vi "BUFMGR_get_maxmem.vi"(11 "error in (no error)":errorcluster) -> (4 "return":u64 format="%.0x", 15 "error out":errorcluster)   [LabVIEW 2016]
uses:
  c/lib/libbuf.so
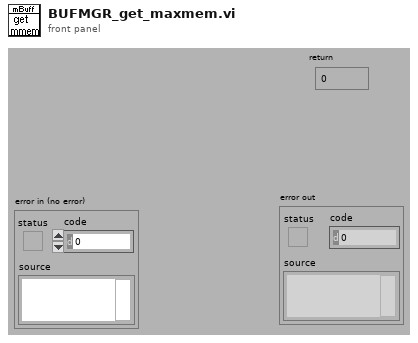
[diagram p1: front panel]
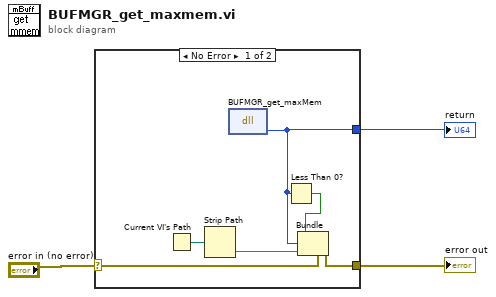
[diagram p0: block diagram]
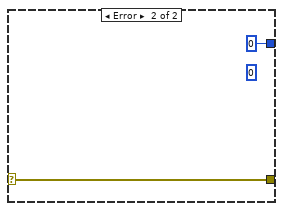
[diagram p2: hidden frame]
diagram:
  n1 = case shown="No Error" "error in (no error)" {
    selector: "error in (no error)" -> [w4 w10]
    tunnel: [w7 u32 0] -> w3
    tunnel: [w9 w10] -> w2
    frame No Error {
      n2 = Current VI's Path() -> (path=w6:path)
      n3 = Strip Path(path=w6) -> (name=w5:string)  [unwired: 1 out]
      n4 = dll-call lib="home/simager/panview/PAN/Modules/buffermgr/private/c/lib/libbuf.so" fn="BUFMGR_get_maxMem"() -> ("return type"=w7:u64)  [unwired: 3 in, 2 out]
      n5 = Less Than 0?(x=w7) -> (x < 0?=w8:bool)
      n6 = Bundle(cluster=w4, "status"=w8, "code"=w7, "source"=w5) -> (w9:errorcluster)
    }
    frame Error {
      (unwired) 0 ("size")
    }
  }
  "error out" <- w2
  "return" <- w3
